vi "Update Controller Settings on Delete.vi"(8 "error in (no error)":errorcluster, 11 "Item Ref in":T1 format="%.0x") -> (0 "error out":errorcluster, 3 "Item Ref out":T1 format="%.0x")   [LabVIEW 2019, in "SEECD System Explorer.lvlib"]
uses:
  SEECD System Explorer.lvlib
  <vilib>/NI VeriStand/Custom Device Tools/Custom Device Utility Library/Custom Device Utility Library.lvlib
  Shared/Globals/Scan Engine GUIDs.vi
  Shared/SEECD Shared.lvlib
  Shared/Type Defs/Host - FPGAScanInterfaceMode.ctl
  <vilib>/NI VeriStand/Custom Device Tools/Custom Device Utility Library/NI VeriStand - Search for Item by GUID.vi
  <vilib>/NI VeriStand/Custom Device API/Custom Device Item Ref.ctl
  <vilib>/NI VeriStand/Custom Device API/Custom Device API.lvlib
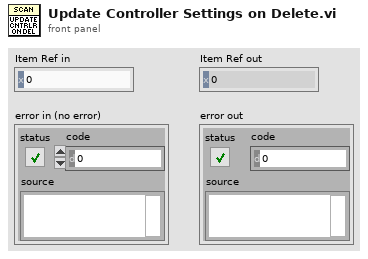
[diagram p1: front panel]
types:
  T1 = typedef "Custom Device API.lvlib/Custom Device Item Ref.ctl" = u64
  T2 = typedef "SEECD Shared.lvlib/Host - FPGAScanInterfaceMode.ctl" = enum16{"Use Current", "FPGA", "Scan Mode"}
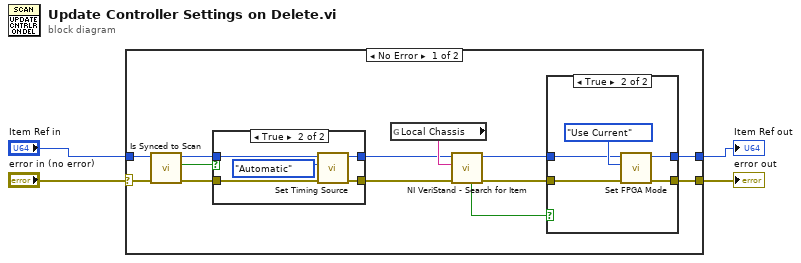
[diagram p0: block diagram]
diagram:
  n1 = case shown="No Error" "error in (no error)" {
    selector: "error in (no error)" -> [w6 w33]
    tunnel: [w17 w32] -> w4
    tunnel: [w16 w33] -> w3
    tunnel: "Item Ref in" -> [w5 w32]
    frame No Error {
      n2 = call "Is Synced to Scan.vi"("error in"=w6, "Item Ref in"=w5) -> ("error out"=w9:errorcluster, "Sync to Scan?"=w7:bool, "Item Ref out"=w8:T1)  [unwired: 6 in, 1 out]
      n3 = case shown="True" w7 {
        tunnel: w8 -> [w25 w31]
        tunnel: w9 -> [w26 w29]
        tunnel: [w26 w28] -> w11
        tunnel: [w25 w27] -> w10
        frame False {
        }
        frame True {
          n4 = call "Set Timing Source.vi"("error in (no error)"=w29, "Timing Source"=enum16{"Automatic", "Custom Device"}."Automatic", "Item Ref in"=w31) -> ("error out"=w28:errorcluster, "Item Ref out"=w27:T1)  [unwired: 7 in]
        }
      }
      n5 = global read "Scan Engine GUIDs.vi" "Local Chassis"() -> (w12:string)
      n6 = call-poly <vilib>:"NI VeriStand - Search for Item.vi"("error in"=w11, "Item GUID"=w12, "Section Ref in"=w10) -> ("error out"=w15:errorcluster, "Section Ref out"=w14:T1, "Found"=w13:bool)  [unwired: 5 in, 1 out]
      n7 = case shown="True" w13 {
        tunnel: w14 -> [w19 w23]
        tunnel: w15 -> [w18 w22]
        tunnel: [w18 w21] -> w16
        tunnel: [w19 w20] -> w17
        frame False {
        }
        frame True {
          n8 = call "Set FPGA Mode.vi"("error in (no error)"=w22, "FPGAScanInterfaceMode"=Host_-_FPGAScanInterfaceMode."Use Current", "Item Ref in"=w23) -> ("error out"=w21:errorcluster, "Item Ref out"=w20:T1)  [unwired: 7 in]
        }
      }
    }
    frame Error {
    }
  }
  "Item Ref out" <- w4
  "error out" <- w3
